vi "Read-Save ObieFile.vi"(6 "Task":enum16{"Save", "Read"}(ring)=enum."Read", 11 "DataPath":path) -> (0 "Pref Path":path, 1 "Success?":bool, 3 "DataPath Out":path)   [LabVIEW 2022 SP3]
panel:
  out "text":string
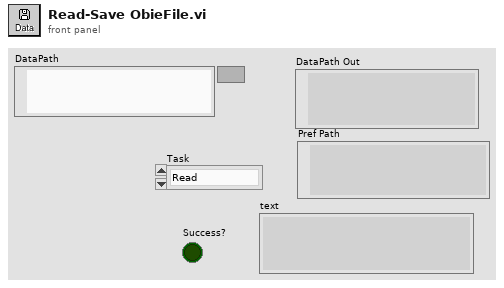
[diagram p1: front panel]
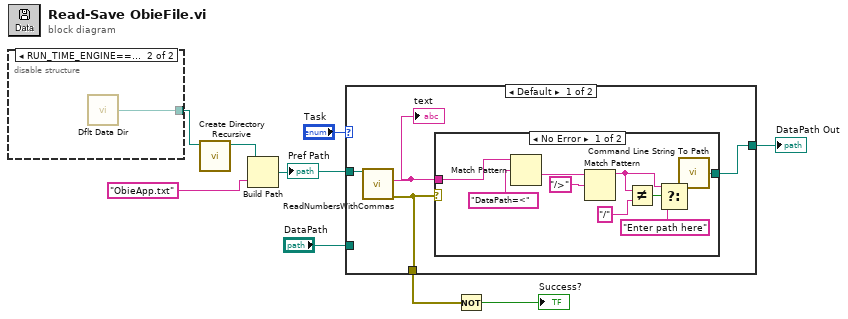
[diagram p0: block diagram]
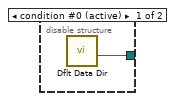
[diagram p2: hidden frame]
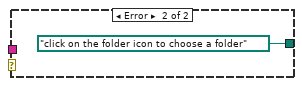
[diagram p3: hidden frame]
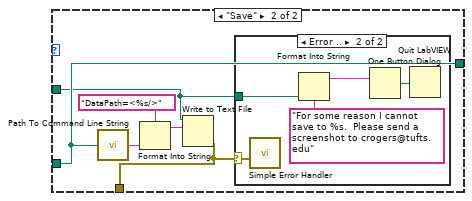
[diagram p4: hidden frame]
diagram:
  n1 = disable-structure shown="RUN_TIME_ENGINE==True" {
    disable-tunnel: [w10 w11] -> w2
    frame condition #0 (active) {
      n2 = call <vilib>:"Dflt Data Dir.vi"() -> ("App:Default Data Directory"=w10:path)
    }
    frame condition #1 {
      n3 = call <vilib>:"Dflt Data Dir.vi"() -> ("App:Default Data Directory"=w11:path)
    }
  }
  n4 = call <vilib>:"Create Directory Recursive.vi"("directory"=w2) -> ("directory copy"=w1:path)  [unwired: 4 in, 2 out]
  n5 = Build Path(base path=w1, name or relative path="ObieApp.txt") -> (appended path=w5:path)
  "Pref Path" <- w5
  n6 = case shown="Default" "Task" {
    tunnel: "DataPath" -> [_ w30]
    tunnel: w5 -> [w14 w27]
    tunnel: [w12 w28] -> w4
    tunnel: [w15 w30] -> w7
    frame Default {
      n7 = call "ReadNumbersWithCommas.vi"("file (use dialog)"=w14) -> ("error out"=w12:errorcluster, "text"=w13:string)  [unwired: 7 in, 2 out]
      "text" <- w13
      n8 = case shown="No Error" w12 {
        tunnel: [w25 path "click on the folder icon to choose a folder" ("path")] -> w15
        tunnel: w13 -> [w24 _]
        frame No Error {
          n9 = Match Pattern(string=w24, regular expression="DataPath=<" ("format string")) -> (after substring=w23:string)  [unwired: 1 in, 3 out]
          n10 = Match Pattern(string=w23, regular expression="/>" ("format string")) -> (before substring=w18:string)  [unwired: 1 in, 3 out]
          n11 = Not Equal?(x=w18, y="/" ("format string")) -> (x != y?=w19:bool)
          n12 = Select(t=w18, s=w19, f="Enter path here" ("format string")) -> (s? t:f=w17:string)
          n13 = call <vilib>:"Command Line String To Path.vi"("string"=w17) -> ("path"=w25:path)
        }
        frame Error {
        }
      }
    }
    frame "Save" {
      n14 = call <vilib>:"Path To Command Line String.vi"("path"=w30) -> ("string"=w29:string)
      n15 = Format Into String(format string="DataPath=<%s/>", w29) -> (resulting string=w32:string)  [unwired: 2 in, 1 out]
      n16 = Write to Text File(file (use dialog)=w27, text=w32) -> (error out=w28:errorcluster)  [unwired: 2 in, 2 out]
      n17 = case shown="Error .." w28 {
        selector: w28 -> [_ w34]
        tunnel: w27 -> [_ w36]
        frame No Error {
        }
        frame Error {
          n18 = call <vilib>:"Simple Error Handler.vi"("error in (no error)"=w34) -> ()  [unwired: 4 in, 5 out]
          n19 = Format Into String(format string="For some reason I cannot save to %s.  Please send a screenshot to crogers@tufts.edu", w36) -> (resulting string=w35:string)  [unwired: 2 in, 1 out]
          n20 = One Button Dialog(message=w35) -> (true=w33:bool)  [unwired: 1 in]
          n21 = Quit LabVIEW(quit? (T)=w33) -> ()
        }
      }
    }
  }
  "DataPath Out" <- w7
  n22 = Not(x=w4) -> (.not. x?=→"Success?":bool)
